vi "test.vi"(8 "error in (no error)":errorcluster) -> (0 "error out":errorcluster, 2 "s? t:f":string, 3 "P/F":bool)   [LabVIEW 2020]
panel:
  in  "stop":bool
  in  "OK Button":bool
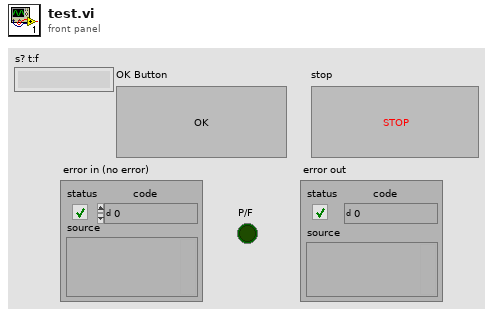
[diagram p1: front panel]
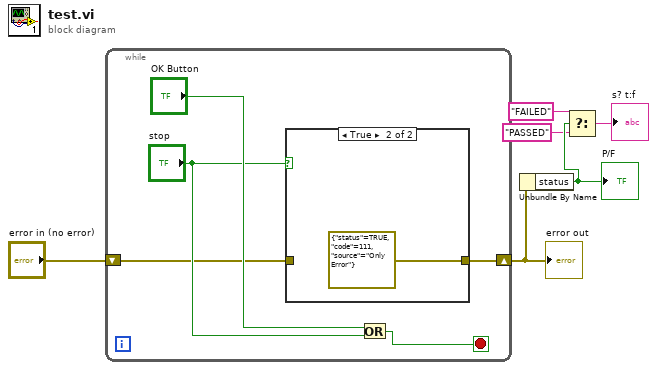
[diagram p0: block diagram]
diagram:
  n1 = while {
    shift-right: [w7] -> w5
    shift-left: "error in (no error)" -> [w8]
    stop <- w10 stop-if-true
    n2 = case shown="True" "stop" {
      tunnel: w8 -> [w12 _]
      tunnel: [w12 errorcluster {"status"=TRUE, "code"=111, "source"="Only Error"} ("error in (no error)")] -> w7
      frame False {
      }
      frame True {
      }
    }
    n3 = Or(x="OK Button", y="stop") -> (x .or. y?=w10:bool)
  }
  "error out" <- w5
  n4 = Unbundle By Name(w5) -> ("status"=w4:bool)
  "P/F" <- w4
  n5 = Select(t="FAILED", s=w4, f="PASSED") -> (s? t:f=→"s? t:f":string)
